vi "SA_AVG.vi"(0 "Session In":refnum<visa-resource-name>="GPIB0::16::INSTR", 1 "Timeout":u32=3000, 2 "IsPSA(t)":bool, 5 "AVG Count":i32=16, 11 "error in":errorcluster {"code" format="%.0x"}, 12 "Trace Type (0: Clear Write)":i32(ring) items=["Clear Write", "Average", "Maximum Hold", "Minimum Hold"], 13 "AVG Restart (T)":bool, 14 "Send OPC? (T)":bool) -> (4 "Session Out":refnum<visa-resource-name>, 15 "error out":errorcluster {"code" format="%.0x"})   [LabVIEW 2018]
doc: "Launches the Instrument I/O Assistant, which you can use to communicate with message-based instruments and graphically parse the response. For example you can communicate with an instrument that uses a serial, Ethernet, or GPIB interface."
uses:
  Initialize References/Station References Global.vi
panel:
  out "String":string
  out "Complete?(t)":bool
  out "AVG_CNT(CMD)":string
  out "AVG_STAT(CMD)":string
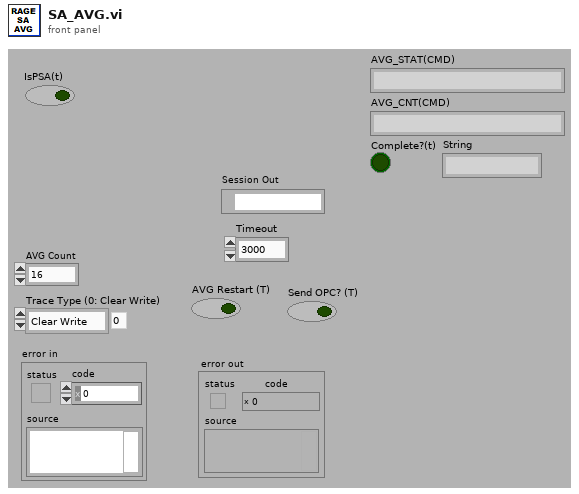
[diagram p1: front panel]
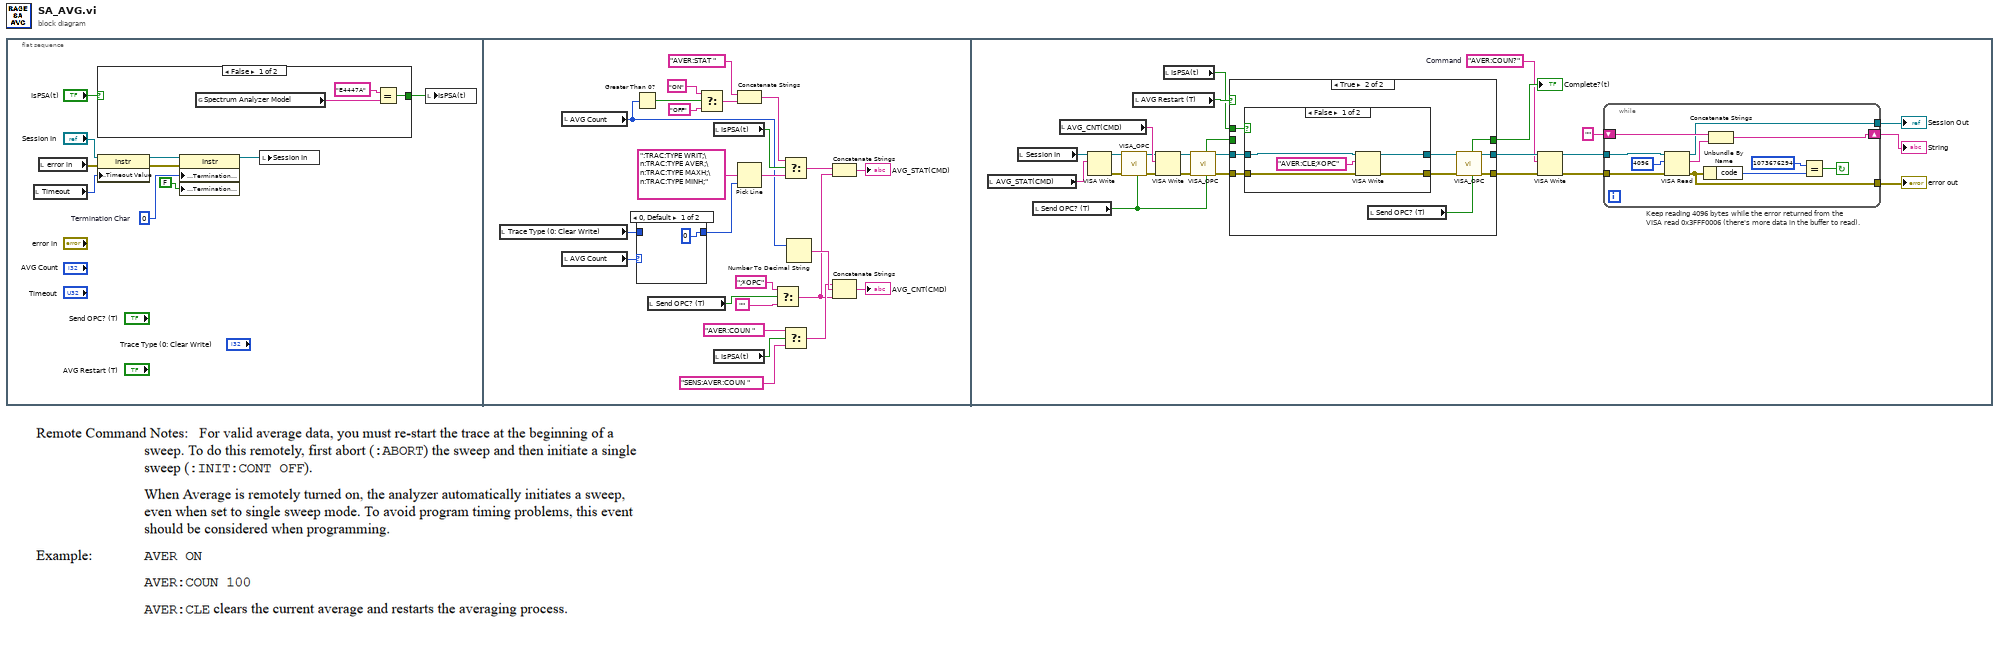
[diagram p0: block diagram]
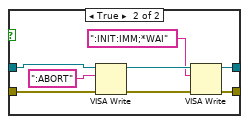
[diagram p5: hidden frame]
diagram:
  n1 = flat-sequence {
    frame #0 {
      w6 = u8 0  # Termination Char
      n2 = local read "Timeout"() -> (w10:u32)
      n3 = local read "error in"() -> (w7:errorcluster)
      n4 = case shown="False" "IsPSA(t)" {
        selector: "IsPSA(t)" -> [_ w14]
        tunnel: [w11 w14] -> w2
        frame False {
          n5 = global read "Station References Global.vi" "Spectrum Analyzer Model"() -> (w13:string)
          n6 = Equal?(x="E4447A", y=w13) -> (x = y?=w11:bool)
        }
        frame True {
        }
      }
      n7 = property class="Instr"(reference="Session In", error in=w7, "General Settings:Timeout Value"=w10) -> (reference out=w8:refnum<visa-resource-name>, error out=w9:errorcluster)
      n8 = property class="Instr"(reference=w8, error in=w9, "Message Based Settings:Termination Character"=w6, "Message Based Settings:Termination Character Enable"=FALSE ("enable")) -> (reference out=w3:refnum<visa-resource-name>)  [unwired: 1 out]
      n9 = local write "Session In"(w3) -> ()
      n10 = local write "IsPSA(t)"(w2) -> ()
    }
    frame #1 {
      n11 = local read "Trace Type (0: Clear Write)"() -> (w39:i32)
      n12 = local read "AVG Count"() -> (w32:i32)
      n13 = local read "AVG Count"() -> (w25:i32)
      n14 = Greater Than 0?(x=w32) -> (x > 0?=w31:bool)
      n15 = case shown="0, Default" w25 {
        tunnel: [0 ("AVG Count") w41] -> w38
        tunnel: w39 -> [_ w41]
        frame 0, Default {
        }
        frame 1.. {
        }
      }
      n16 = local read "Send OPC? (T)"() -> (w16:bool)
      n17 = Select(t="ON" ("staticText"), s=w31, f="OFF" ("staticText")) -> (s? t:f=w29:string)
      n18 = local read "IsPSA(t)"() -> (w33:bool)
      n19 = local read "IsPSA(t)"() -> (w20:bool)
      n20 = Concatenate Strings("AVER:STAT " ("staticText"), w29) -> (w28:string)
      n21 = Pick Line(multi-line string=":TRAC:TYPE WRIT;\n:TRAC:TYPE AVER;\n:TRAC:TYPE MAXH;\n:TRAC:TYPE MINH;", line index=w38) -> (output string=w34:string)  [unwired: 1 in]
      n22 = Select(t=";*OPC" ("staticText"), s=w16, f="") -> (s? t:f=w15:string)
      n23 = Select(t=w28, s=w33, f=w34) -> (s? t:f=w35:string)
      n24 = Select(t="AVER:COUN " ("staticText"), s=w20, f="SENS:AVER:COUN " ("staticText")) -> (s? t:f=w22:string)
      n25 = Number To Decimal String(number=w32) -> (decimal integer string=w37:string)  [unwired: 1 out]
      n26 = Concatenate Strings(w35, w15) -> (→"AVG_STAT(CMD)":string)
      n27 = Concatenate Strings(w22, w37, w15) -> (→"AVG_CNT(CMD)":string)
    }
    frame #2 {
      w46 = "AVER:COUN?"  # Command
      # "Keep reading 4096 bytes while the error returned from the\nVISA read 0x3FFF0006 (there's more data in the buffer to read)."
      n28 = local read "AVG_STAT(CMD)"() -> (w66:string)
      n29 = local read "Session In"() -> (w44:refnum<visa-resource-name>)
      n30 = local read "Send OPC? (T)"() -> (w50:bool)
      n31 = local read "AVG_CNT(CMD)"() -> (w65:string)
      n32 = VISA Write(VISA resource name=w44, write buffer=w66) -> (VISA resource name out=w59:refnum<visa-resource-name>, error out=w56:errorcluster)  [unwired: 1 in, 1 out]
      n33 = call "VISA_OPC.vi"("OPC(T)"=w50, "error in"=w56, "Session In"=w59) -> ("error out"=w57:errorcluster, "Session Out"=w58:refnum<visa-resource-name>)  [unwired: 6 in, 1 out]
      n34 = local read "AVG Restart (T)"() -> (w64:bool)
      n35 = VISA Write(VISA resource name=w58, write buffer=w65, error in (no error)=w57) -> (VISA resource name out=w61:refnum<visa-resource-name>, error out=w60:errorcluster)  [unwired: 1 out]
      n36 = local read "IsPSA(t)"() -> (w42:bool)
      n37 = call "VISA_OPC.vi"("OPC(T)"=w50, "error in"=w60, "Session In"=w61) -> ("error out"=w62:errorcluster, "Session Out"=w63:refnum<visa-resource-name>, "OPC?(T)"=w43:bool)  [unwired: 6 in]
      n38 = case shown="True" w64 {
        tunnel: w62 -> [w79 w89]
        tunnel: [w79 w87] -> w52
        tunnel: w63 -> [w80 w88]
        tunnel: [w80 w84] -> w53
        tunnel: [w78 w82] -> w51
        tunnel: w43 -> [w78 _]
        tunnel: w42 -> [_ w81]
        frame False {
        }
        frame True {
          n39 = case shown="False" w81 {
            tunnel: w89 -> [w94 w95]
            tunnel: w88 -> [w93 w96]
            tunnel: [w92 w98] -> w86
            tunnel: [w91 w97] -> w85
            frame False {
              n40 = VISA Write(VISA resource name=w93, write buffer="AVER:CLE;*OPC" ("StaticText"), error in (no error)=w94) -> (VISA resource name out=w91:refnum<visa-resource-name>, error out=w92:errorcluster)  [unwired: 1 out]
            }
            frame True {
              n41 = VISA Write(VISA resource name=w96, write buffer=":ABORT", error in (no error)=w95) -> (VISA resource name out=w101:refnum<visa-resource-name>, error out=w102:errorcluster)  [unwired: 1 out]
              n42 = VISA Write(VISA resource name=w101, write buffer=":INIT:IMM;*WAI", error in (no error)=w102) -> (VISA resource name out=w97:refnum<visa-resource-name>, error out=w98:errorcluster)  [unwired: 1 out]
            }
          }
          n43 = local read "Send OPC? (T)"() -> (w83:bool)
          n44 = call "VISA_OPC.vi"("OPC(T)"=w83, "error in"=w86, "Session In"=w85) -> ("error out"=w87:errorcluster, "Session Out"=w84:refnum<visa-resource-name>, "OPC?(T)"=w82:bool)  [unwired: 6 in]
        }
      }
      "Complete?(t)" <- w51
      n45 = VISA Write(VISA resource name=w53, write buffer=w46, error in (no error)=w52) -> (VISA resource name out=w49:refnum<visa-resource-name>, error out=w48:errorcluster)  [unwired: 1 out]
      n46 = while {
        tunnel: w49 -> [w74]
        shift-right: [w68] -> w45
        shift-left: "" -> [w73]
        tunnel: w48 -> [w71]
        tunnel: [w70] -> w55
        tunnel: [w67] -> w54
        stop <- w69 continue-if-true
        n47 = VISA Read(VISA resource name=w74, byte count=u32 4096 ("byte count (0)"), error in (no error)=w71) -> (VISA resource name out=w67:refnum<visa-resource-name>, read buffer=w72:string, error out=w70:errorcluster)  [unwired: 1 out]
        n48 = Unbundle By Name(w70) -> ("code"=w76:i32)
        n49 = Concatenate Strings(w73, w72) -> (w68:string)
        n50 = Equal?(x=1073676294, y=w76) -> (x = y?=w69:bool)
      }
      "error out" <- w55
      "Session Out" <- w54
      "String" <- w45
    }
  }
